vi "Cub Meaasure FGV.vi"(0 "Action":T1=enum."Write", 1 "AddTable 6":string[][](table)=[["Tray Barcode", ""], ["PCBA BARCODE", ""], ["硬體(Tool初始化)", ""], ["company(Tool初始化)", ""], ["耗電流 uA(電流表)", ""], ["電池負載電壓", ""], ["晶片ID(Tool FORMAT)", ""], ["雷雕ID(TOOl scan、藍芽接收器)", ""], ["Format(Tool FORMAT)", ""], ["Programe(Tool Programe)", ""], ["MAC(藍芽接收器)", ""], ["ID(藍芽接收器)", ""], ["KPA(藍芽接收器)", ""], ["溫度(藍芽接收器)", ""], ["SENSOR電池電壓(藍芽接收器)", ""], ["RSSI(藍芽接收器)", ""], ["SensorType_315(FSK scan)", ""], ["FSKsnVol_315(FSK scan)", ""], ["FSKscanl_315(FSK scan)", ""], ["P_315(Tool FSK scan)", ""], ["T_315(Tool FSK scan)", ""], ["SensorType_433(ASK scan)", ""], ["ASKsnVol_433(ASK scan)", ""], ["ASKscan_433(ASK scan)", ""], ["P_433(ASK scan)", ""], ["T_433(ASK scan)", ""], ["測高Data", ""]], 3 "Save Index":T2=enum."硬體(Tool初始化)", 4 "DataIn":string, 5 "SN":string, 6 "Table Load":cluster{"Table Control":string[][]}[](array[cluster]), 7 "error in (no error)":errorcluster) -> (12 "條碼的Index":i32, 13 "Read SN Table":string[][](array[string]), 14 "Total Table":cluster{"Table Control":string[][]}[](array[cluster]), 15 "Barcode Array":string[](array[string]), 16 "Read Index Data":string, 17 "Read first table":string[][](array[string]), 18 "Barcode重複":bool, 19 "error out":errorcluster)   [LabVIEW 2019]
uses:
  Ctrl/MeasureDisplayTab.ctl
  Ctrl/Table Save.ctl
  9377167a-9215-4fe1-b1d7-405c4c1bac97.vi
  09652be0-0e8a-482c-be89-5823cf7997f4.vi
  <vilib>/Utility/xml.llb/Write to XML File(string).vi
  <vilib>/Utility/xml.llb/Read From XML File(string).vi
panel:
  in  "AddTable 2":string[][](table)=[["PCBA BARCODE", ""], ["硬體(Tool初始化)", ""], ["company(Tool初始化)", ""], ["耗電流 uA(電流表)", ""], ["電池負載電壓", ""], ["晶片ID(Tool FORMAT)", ""], ["雷雕ID(TOOl scan、藍芽接收器)", ""], ["Format(Tool FORMAT)", ""], ["Programe(Tool Programe)", ""], ["MAC(藍芽接收器)", ""], ["ID(藍芽接收器)", ""], ["KPA(藍芽接收器)", ""], ["溫度(藍芽接收器)", ""], ["SENSOR電池電壓(藍芽接收器)", ""], ["RSSI(藍芽接收器)", ""], ["SensorType_315(FSK scan)", ""], ["FSKsnVol_315(FSK scan)", ""], ["FSKscanl_315(FSK scan)", ""], ["P_315(Tool FSK scan)", ""], ["T_315(Tool FSK scan)", ""], ["SensorType_433(ASK scan)", ""], ["ASKsnVol_433(ASK scan)", ""], ["ASKscan_433(ASK scan)", ""], ["P_433(ASK scan)", ""], ["T_433(ASK scan)", ""], ["測高Data", ""]]
  in  "WriteTable":string[][](table)=[["PCBA BARCODE", ""], ["硬體(Tool初始化)", ""], ["company(Tool初始化)", ""], ["耗電流 uA(電流表)", ""], ["電池負載電壓", ""], ["晶片ID(Tool FORMAT)", ""], ["雷雕ID(TOOl scan、藍芽接收器)", ""], ["Format(Tool FORMAT)", ""], ["Programe(Tool Programe)", ""]]
  out "index of element":i32
  out "LOG":string[][](array[string])
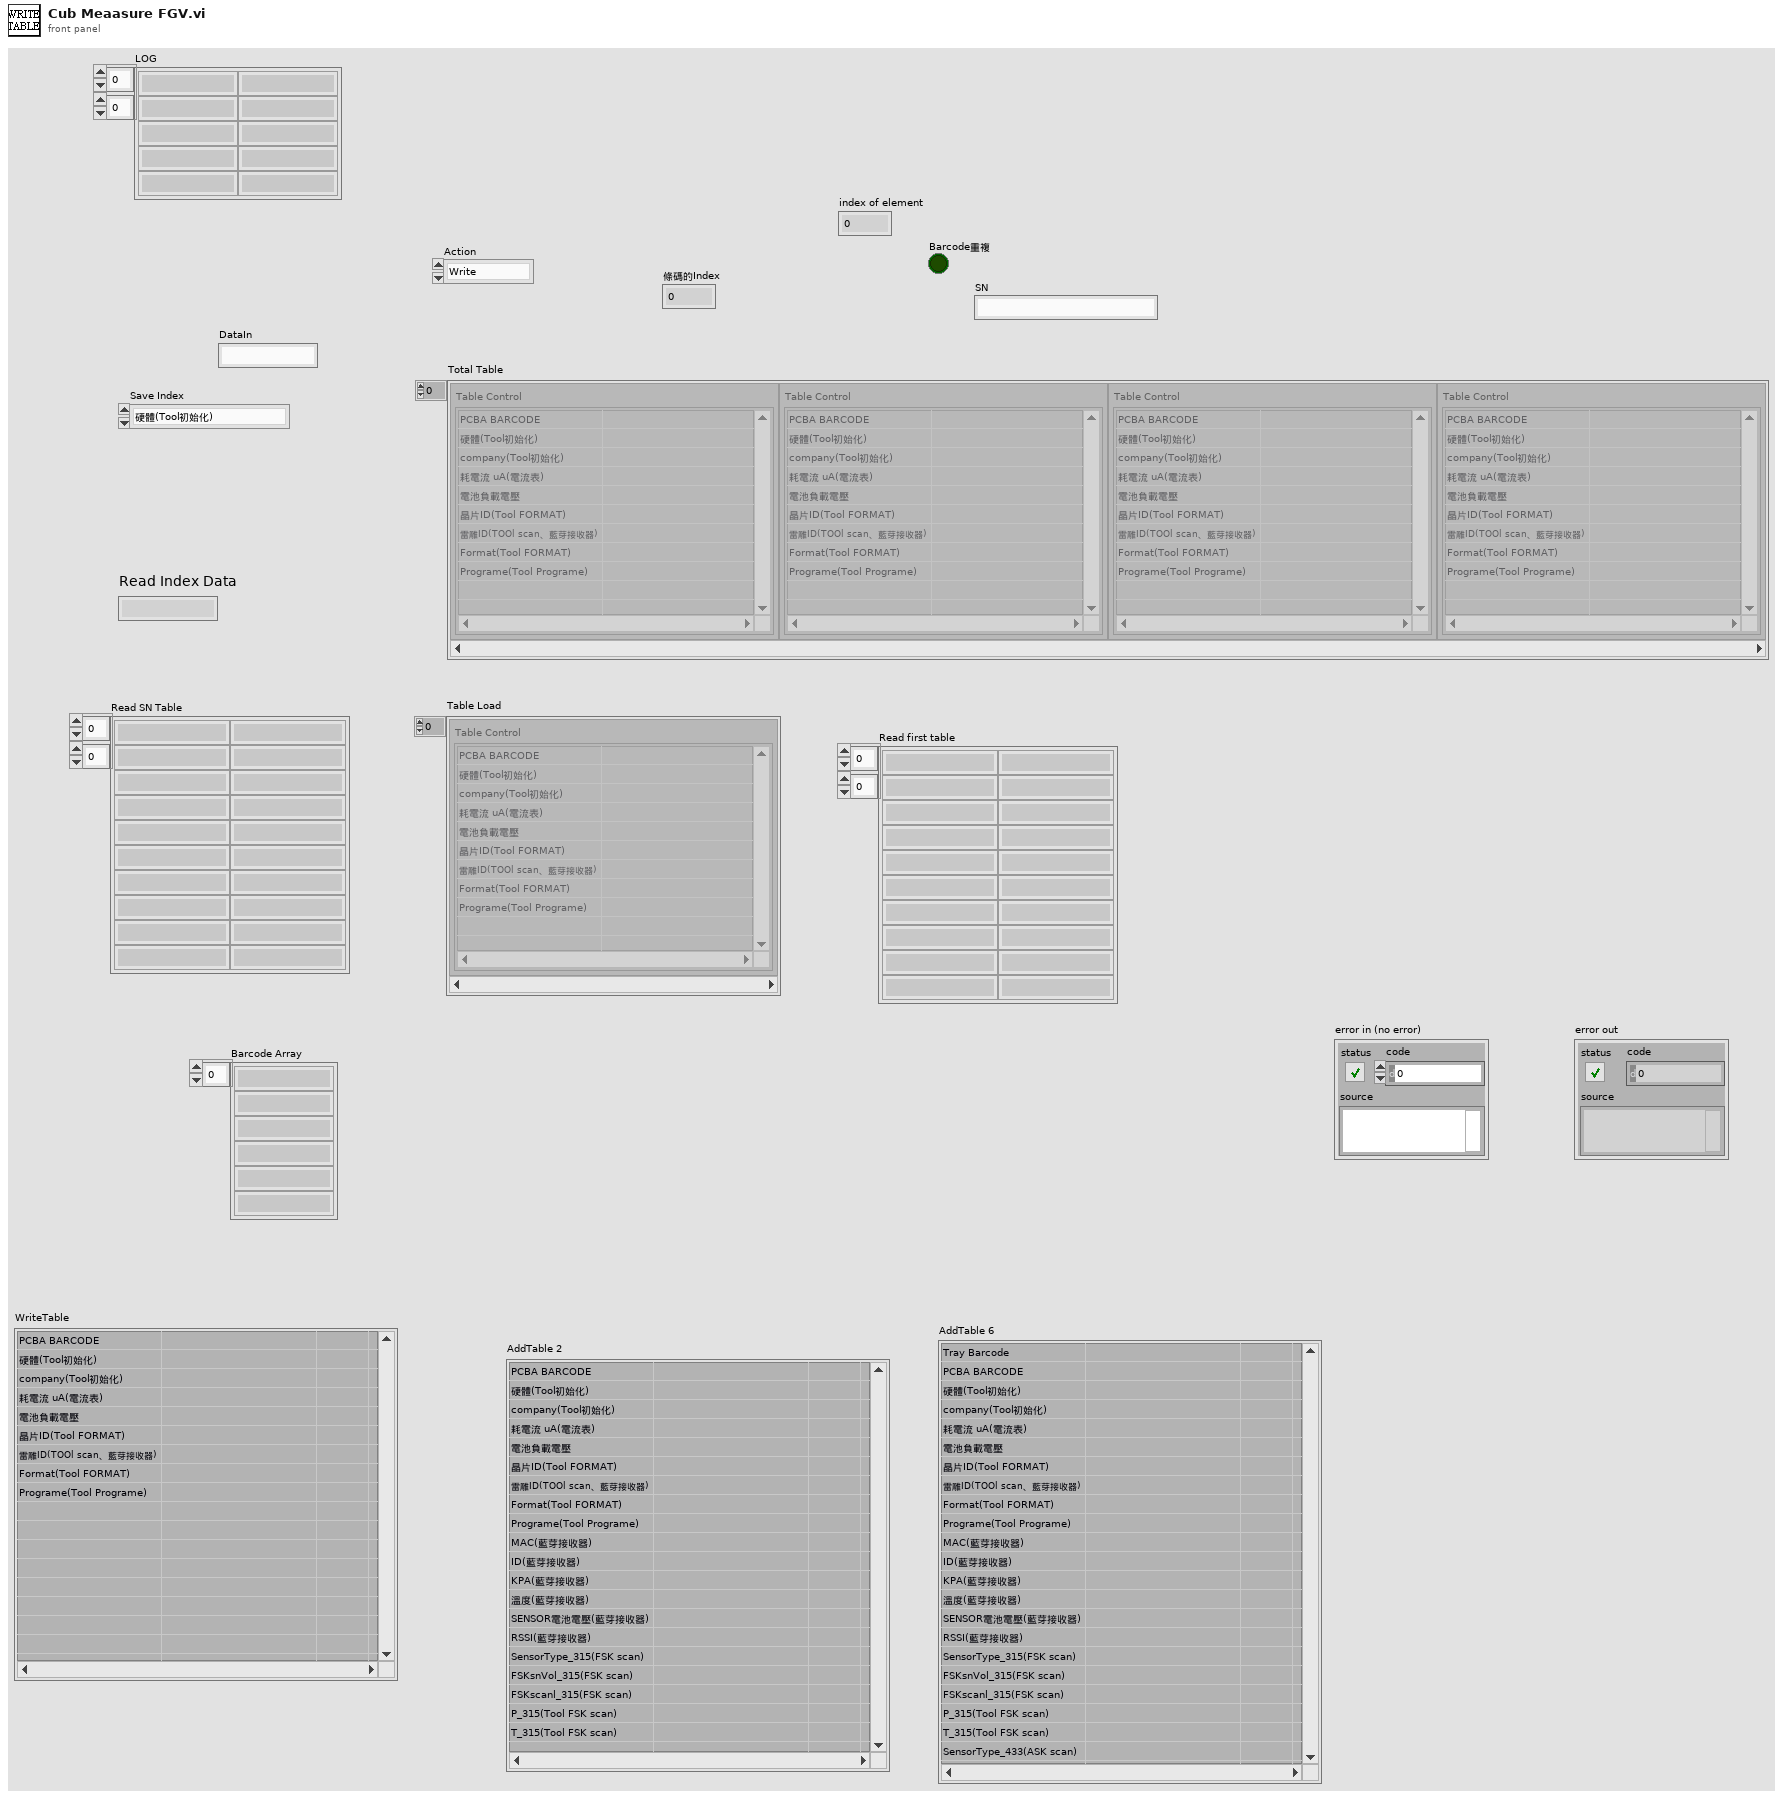
[diagram p1: front panel]
types:
  T1 = typedef "Table Save.ctl" = enum16{"initial", "Add", "Write", "Replace", "Delete", "REad", "RedTable", "Load"}
  T2 = typedef "MeasureDisplayTab.ctl" = enum16{"Tray Barcode", "PCBA BARCODE", "硬體(Tool初始化)", "company(Tool初始化)", "耗電流 uA(電流表)", "電池負載電壓", "晶片ID(Tool FORMAT)", "雷雕ID(TOOl scan、藍芽接收器)", "Format(Tool FORMAT)", "Programe(Tool Programe)", "MAC(藍芽接收器)", "ID(藍芽接收器)", "KPA(藍芽接收器)", "溫度(藍芽接收器)", "SENSOR電池電壓(藍芽接收器)", "RSSI(藍芽接收器)", "SensorType_315(FSK scan)", "FSKsnVol_315(FSK scan)", "FSKscanl_315(FSK scan)", "P_315(FSK scan)", "T_315(FSK scan)", "SensorType_433(ASK scan)", "ASKsnVol_433(ASK scan)", "ASKscan_433(ASK scan)", "P_433(ASK scan)", "T_433(ASK scan)", "測高Data"}
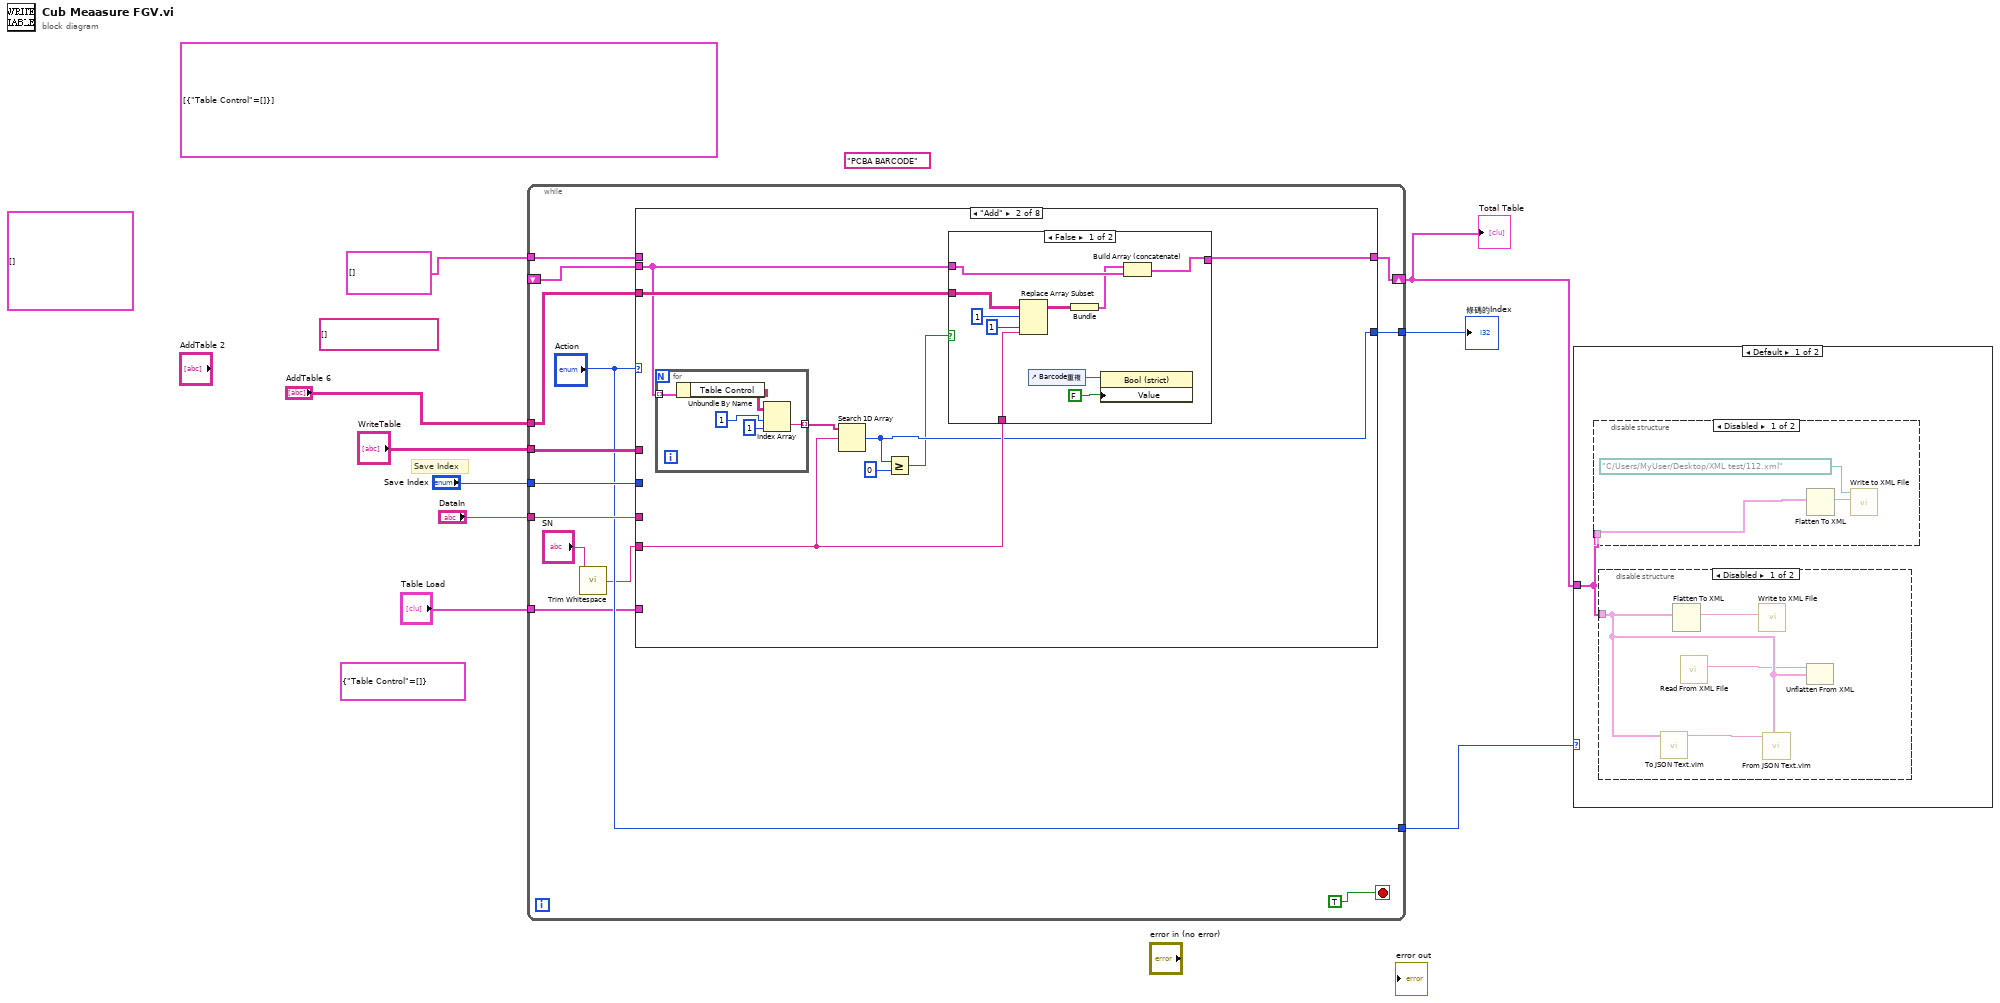
[diagram p0: block diagram]
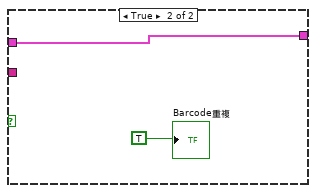
[diagram p6: hidden frame]
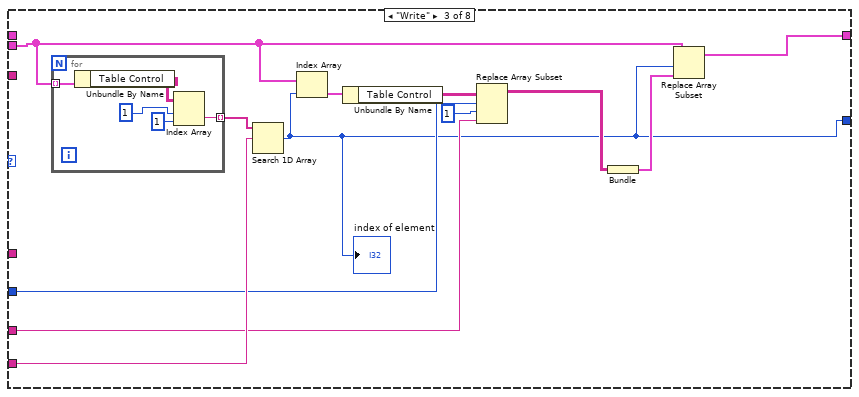
[diagram p7: hidden frame]
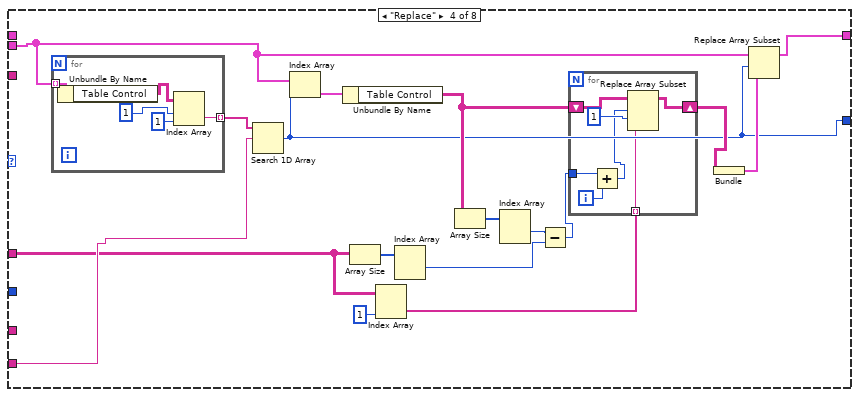
[diagram p8: hidden frame]
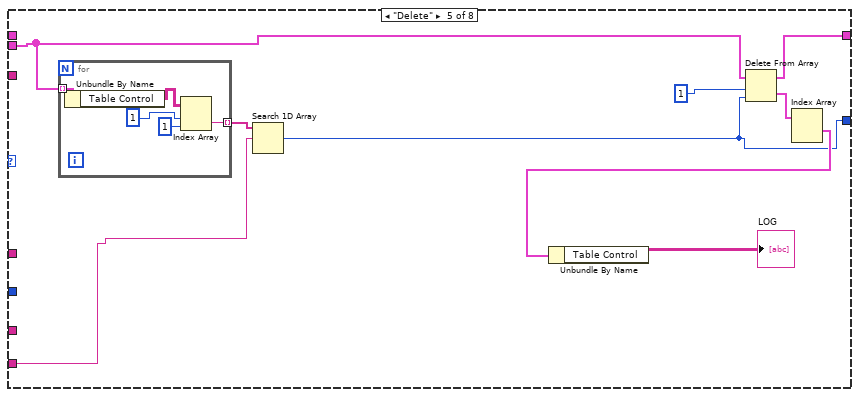
[diagram p9: hidden frame]
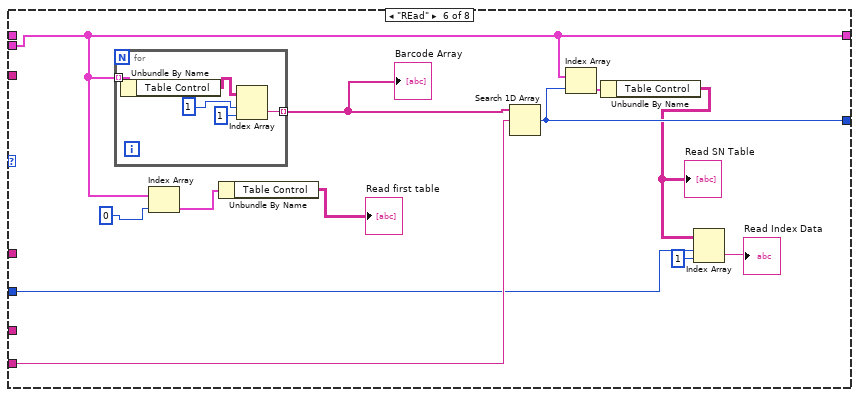
[diagram p10: hidden frame]
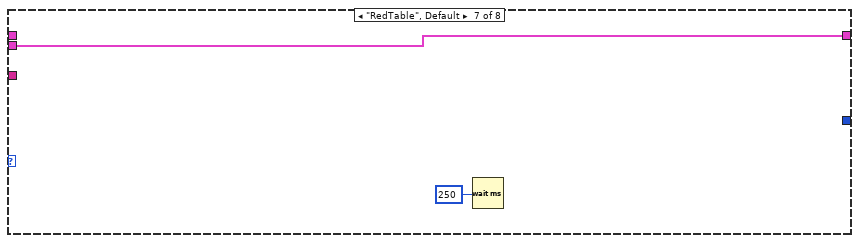
[diagram p11: hidden frame]
diagram:
  (unwired) cluster{"Table Control":string[][]}[] [] ("EnfMeasureTable 2")
  (unwired) cluster{"Table Control":string[][]} {"Table Control"=[]} ("Cluster")
  (unwired) "PCBA BARCODE"
  (unwired) string[][] [] ("Table Control")
  (unwired) cluster{"Table Control":string[][]}[] [{"Table Control"=[]}] ("Array 2")
  # "Save Index"
  n1 = while {
    tunnel: cluster{"Table Control":string[][]}[] [] ("Total Table") -> [w22]
    shift-right: [w21] -> w3
    shift-left: _ -> [w20]
    tunnel: "AddTable 6" -> [w19]
    tunnel: "WriteTable" -> [w16]
    tunnel: ["Action"] -> w8
    tunnel: "Save Index" -> [w18]
    tunnel: "DataIn" -> [w17]
    tunnel: [w14] -> w5
    tunnel: "Table Load" -> [w12]
    stop <- TRUE stop-if-true
    n2 = call <vilib>:"Trim Whitespace.vi"("string"="SN") -> ("trimmed string"=w10:string)  [unwired: 1 in]
    n3 = case shown="\"Add\"" "Action" {
      tunnel: w22 -> [w23 _ _ _ _ _ _ _]
      tunnel: [w23 w31 w59 w80 w96 w118 w127 w128] -> w21
      tunnel: w19 -> [_ w29 _ _ _ _ _ _]
      tunnel: w20 -> [_ w27 w55 w78 w98 w118 w127 _]
      tunnel: w10 -> [_ w28 w57 w77 w102 w119 _ _]
      tunnel: w18 -> [_ _ w51 _ _ w111 _ _]
      tunnel: w17 -> [_ _ w50 _ _ _ _ _]
      tunnel: w16 -> [_ _ _ w67 _ _ _ _]
      tunnel: [_ w26 w49 w66 w95 w116 _ _] -> w14
      tunnel: w12 -> [_ _ _ _ _ _ _ w128]
      frame "initial" {
      }
      frame "Add" {
        n4 = for {
          tunnel: w27 -> [w48] mode=indexing
          tunnel: [w44] -> w30 mode=indexing
          n5 = Unbundle By Name(w48) -> ("Table Control"=w47:string[][])
          n6 = Index Array(array=w47, index (row)=1 ("disabled index (col)"), index (col)=1 ("disabled index (col)")) -> (element=w44:string)
        }
        n7 = Search 1D Array(1D array=w30, element=w28) -> (index of element=w26:i32)  [unwired: 1 in]
        n8 = Greater Or Equal?(x=w26, y=0) -> (x >= y?=w24:bool)
        n9 = case shown="False" w24 {
          tunnel: [w41 w43] -> w31
          tunnel: w29 -> [w38 _]
          tunnel: w28 -> [w37 _]
          tunnel: w27 -> [w33 w43]
          frame False {
            n10 = Replace Array Subset(array=w38, new element=w37, index (row)=1, index (col)=1) -> (w34:string[][])
            n11 = control-ref of="Barcode重複"() -> (w36:refnum<vi>)
            n12 = Bundle("AddTable 6"=w34) -> (w32:cluster{"AddTable 6":string[][]})  [unwired: 1 in]
            n13 = property class="Bool (strict)"(reference=w36, "Value"=FALSE) -> ()  [unwired: 1 in, 2 out]
            n14 = Build Array (concatenate)(w32, w33) -> (w41:cluster{"Table Control":string[][]}[])
          }
          frame True {
            "Barcode重複" <- TRUE
          }
        }
      }
      frame "Write" {
        n15 = for {
          tunnel: w55 -> [w65] mode=indexing
          tunnel: [w61] -> w60 mode=indexing
          n16 = Unbundle By Name(w65) -> ("Table Control"=w64:string[][])
          n17 = Index Array(array=w64, index (row)=1 ("disabled index (col)"), index (col)=1 ("disabled index (col)")) -> (element=w61:string)
        }
        n18 = Search 1D Array(1D array=w60, element=w57) -> (index of element=w49:i32)  [unwired: 1 in]
        "index of element" <- w49
        n19 = Index Array(array=w55, index=w49) -> (element=w56:cluster{"Table Control":string[][]})
        n20 = Unbundle By Name(w56) -> ("Table Control"=w54:string[][])
        n21 = Replace Array Subset(array=w54, new element=w50, index (row)=w51, index (col)=1) -> (w52:string[][])
        n22 = Bundle("Table Control"=w52) -> (w58:cluster{"Table Control":string[][]})  [unwired: 1 in]
        n23 = Replace Array Subset(array=w55, new element=w58, index=w49) -> (w59:cluster{"Table Control":string[][]}[])
      }
      frame "Replace" {
        n24 = for {
          tunnel: w78 -> [w94] mode=indexing
          tunnel: [w90] -> w82 mode=indexing
          n25 = Unbundle By Name(w94) -> ("Table Control"=w93:string[][])
          n26 = Index Array(array=w93, index (row)=1 ("disabled index (col)"), index (col)=1 ("disabled index (col)")) -> (element=w90:string)
        }
        n27 = Search 1D Array(1D array=w82, element=w77) -> (index of element=w66:i32)  [unwired: 1 in]
        n28 = Index Array(array=w78, index=w66) -> (element=w81:cluster{"Table Control":string[][]})
        n29 = Unbundle By Name(w81) -> ("Table Control"=w70:string[][])
        n30 = Array Size(array=w67) -> (size(s)=w74:i32[])
        n31 = Index Array(array=w67, index (col)=1 ("disabled index (col)")) -> (element=w71:string[])  [unwired: 1 in]
        n32 = Index Array(array=w74) -> (element #1=w73:i32)  [unwired: 2 in, 1 out]
        n33 = Array Size(array=w70) -> (size(s)=w75:i32[])
        n34 = Index Array(array=w75) -> (element #1=w69:i32)  [unwired: 2 in, 1 out]
        n35 = Subtract(x=w69, y=w73) -> (x-y=w68:i32)
        n36 = for {
          shift-right: [w89] -> w76
          shift-left: w70 -> [w88]
          tunnel: w68 -> [w85]
          tunnel: w71 -> [w84] mode=indexing
          i -> [w86]
          n37 = Add(x=w85, y=w86) -> (x+y=w83:i32)
          n38 = Replace Array Subset(array=w88, new element=w84, index (row)=w83, index (col)=1 ("disabled index (col)")) -> (w89:string[][])
        }
        n39 = Bundle("Table Control"=w76) -> (w79:cluster{"Table Control":string[][]})  [unwired: 1 in]
        n40 = Replace Array Subset(array=w78, new element=w79, index=w66) -> (w80:cluster{"Table Control":string[][]}[])
      }
      frame "Delete" {
        n41 = for {
          tunnel: w98 -> [w108] mode=indexing
          tunnel: [w104] -> w103 mode=indexing
          n42 = Unbundle By Name(w108) -> ("Table Control"=w107:string[][])
          n43 = Index Array(array=w107, index (row)=1 ("disabled index (col)"), index (col)=1 ("disabled index (col)")) -> (element=w104:string)
        }
        n44 = Search 1D Array(1D array=w103, element=w102) -> (index of element=w95:i32)  [unwired: 1 in]
        n45 = Delete From Array(array=w98, length=1 ("index"), index=w95) -> (deleted portion=w101:cluster{"Table Control":string[][]}[], array with subset deleted=w96:cluster{"Table Control":string[][]}[])
        n46 = Index Array(array=w101) -> (element #1=w100:cluster{"Table Control":string[][]})  [unwired: 2 in, 1 out]
        n47 = Unbundle By Name(w100) -> ("Table Control"=→"LOG":string[][])
      }
      frame "REad" {
        n48 = for {
          tunnel: w118 -> [w125] mode=indexing
          tunnel: [w121] -> w120 mode=indexing
          n49 = Unbundle By Name(w125) -> ("Table Control"=w124:string[][])
          n50 = Index Array(array=w124, index (row)=1 ("disabled index (col)"), index (col)=1 ("disabled index (col)")) -> (element=w121:string)
        }
        "Barcode Array" <- w120
        n51 = Index Array(array=w118, index=0) -> (element=w115:cluster{"Table Control":string[][]})
        n52 = Unbundle By Name(w115) -> ("Table Control"=→"Read first table":string[][])
        n53 = Search 1D Array(1D array=w120, element=w119) -> (index of element=w116:i32)  [unwired: 1 in]
        n54 = Index Array(array=w118, index=w116) -> (element=w117:cluster{"Table Control":string[][]})
        n55 = Unbundle By Name(w117) -> ("Table Control"=w112:string[][])
        "Read SN Table" <- w112
        n56 = Index Array(array=w112, index (row)=w111, index (col)=1 ("disabled index (col)")) -> (element=→"Read Index Data":string)
      }
      frame "RedTable", Default {
        n57 = Wait (ms)(milliseconds to wait=250) -> ()  [unwired: 1 out]
      }
      frame "Load" {
      }
    }
  }
  "條碼的Index" <- w5
  "Total Table" <- w3
  n58 = case shown="Default" w8 {
    tunnel: w3 -> [w129 _]
    frame Default {
      n59 = disable-structure shown="Disabled" {
        disable-tunnel: w129 -> [w130 _]
        frame Disabled {
          n60 = Flatten To XML(anything=w130) -> (xml string=w132:string)
          n61 = call-poly <vilib>:"Write to XML File.vi"("XML Input"=w132, "XML File Path"=path "C:/Users/MyUser/Desktop/XML test/112.xml") -> ()  [unwired: 7 in, 3 out]
        }
        frame Enabled {
        }
      }
      n62 = disable-structure shown="Disabled" {
        disable-tunnel: w129 -> [w135 _]
        frame Disabled {
          n63 = call "To JSON Text.vim"("Anything"=w135) -> ("<JSON>"=w136:string)  [unwired: 9 in, 1 out]
          n64 = Flatten To XML(anything=w135) -> (xml string=w133:string)
          n65 = call-poly <vilib>:"Read From XML File.vi"() -> ("XML Elements"=w134:string)  [unwired: 9 in, 2 out]
          n66 = call-poly <vilib>:"Write to XML File.vi"("XML Input"=w133) -> ()  [unwired: 8 in, 3 out]
          n67 = call "From JSON Text.vim"("Data Type and Default Value"=w135, "JSON"=w136) -> ()  [unwired: 8 in, 2 out]
          n68 = Unflatten From XML(xml string=w134, type=w135) -> ()  [unwired: 1 in, 2 out]
        }
        frame Enabled {
        }
      }
    }
    frame "initial", "REad" {
    }
  }
